vi "Joystick Outputs w Rumble.vi"(3 "Right Rumble":sgl, 4 "Left Rumble":sgl, 5 "JoystickDevRef":T1) -> (0 "POV":cluster{"POV":i16}, 1 "Axis":T3, 2 "Buttons":T4)   [LabVIEW 2020]
uses:
  <vilib>/Rock Robotics/WPI/Joystick/WPI_JoystickDevRef.ctl
  <vilib>/Rock Robotics/WPI/Joystick/WPI_JoystickDeviceEnum.ctl
panel:
  out "POV BL":bool
  out "POV BR":bool
  out "POV TR":bool
  out "POV TR":bool
  out "POV B":bool
  out "POV T":bool
  out "POV L":bool
  out "POV R":bool
  out "POV C":bool
  out "\"x' 13":bool
  out "\"x' 12":bool
  out "\"x' 11":bool
  out "\"x' 10":bool
  out "\"x' 9":bool
  out "\"x' 8":bool
  out "\"x' 7":bool
  out "\"x' 2":bool
  out "\"x' 6":bool
  out "\"x' 4":bool
  out "\"x' 3":bool
  out "\"x' 2":bool
  out "\"x'":bool
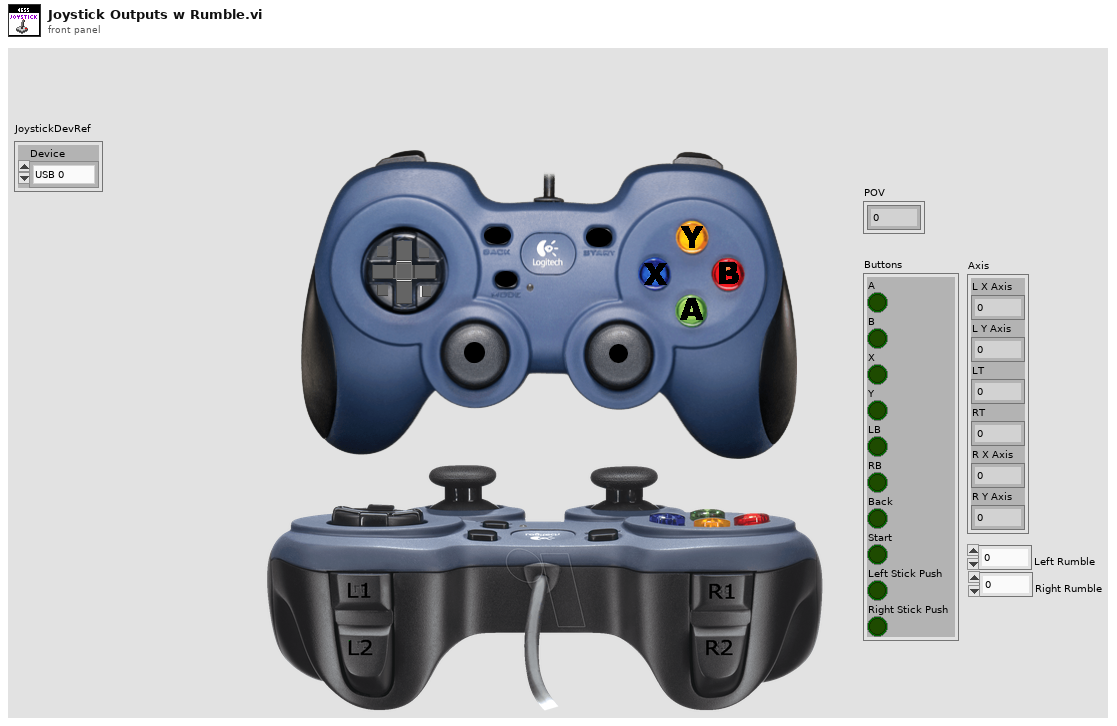
[diagram p1: front panel]
types:
  T1 = typedef "WPI_JoystickDevRef.ctl" = cluster{"Device":T2}
  T2 = typedef "WPI_JoystickDeviceEnum.ctl" = enum16{"USB 0", "USB 1", "USB 2", "USB 3", "USB 4", "USB 5"}
  T3 = cluster{"L X Axis":dbl, "L Y Axis":dbl, "LT":dbl, "RT":dbl, "R X Axis":dbl, "R Y Axis":dbl}
  T4 = cluster{"A":bool, "B":bool, "X":bool, "Y":bool, "LB":bool, "RB":bool, "Back":bool, "Start":bool, "Left Stick Push":bool, "Right Stick Push":bool}
  T5 = cluster{"Buttons[0]":bool, "Buttons[1]":bool, "Buttons[2]":bool, "Buttons[3]":bool, "Buttons[4]":bool, "Buttons[5]":bool, "Buttons[6]":bool, "Buttons[7]":bool, "Buttons[8]":bool, "Buttons[9]":bool}
  T6 = cluster{"Axes[0]":dbl, "Axes[1]":dbl, "Axes[2]":dbl, "Axes[3]":dbl, "Axes[4]":dbl, "Axes[5]":dbl}
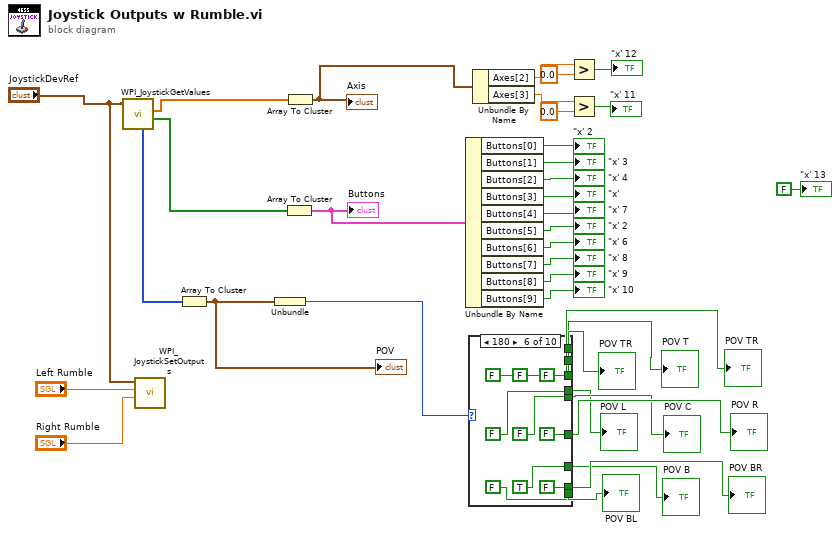
[diagram p0: block diagram]
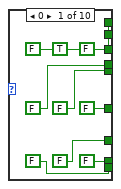
[diagram p2: hidden frame]
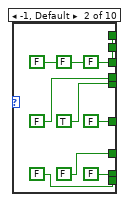
[diagram p3: hidden frame]
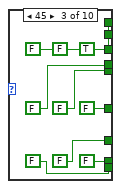
[diagram p4: hidden frame]
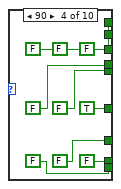
[diagram p5: hidden frame]
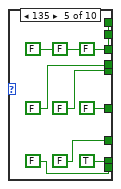
[diagram p6: hidden frame]
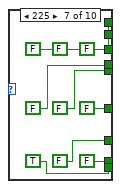
[diagram p7: hidden frame]
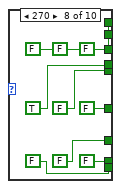
[diagram p8: hidden frame]
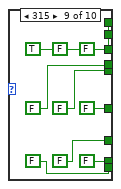
[diagram p9: hidden frame]
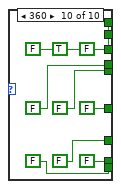
[diagram p10: hidden frame]
diagram:
  n1 = call <vilib>:"WPI_JoystickGetValues.vi"("JoystickDevRef"="JoystickDevRef") -> ("Buttons"=w36:bool[], "Axes"=w35:dbl[], "POVs"=w34:i16[])  [unwired: 6 in, 2 out]
  n2 = call <vilib>:"WPI_JoystickSetOutputs.vi"("Right Rumble"="Right Rumble", "Left Rumble"="Left Rumble", "JoystickDevRef"="JoystickDevRef") -> ()  [unwired: 7 in, 2 out]
  n3 = Array To Cluster(array=w34) -> (cluster=w16:cluster{"POVs[0]":i16})
  "POV" <- w16
  n4 = Unbundle(w16) -> ("POVs[0]"=w5:i16)
  n5 = Array To Cluster(array=w36) -> (cluster=w33:T5)
  "Buttons" <- w33
  n6 = Array To Cluster(array=w35) -> (cluster=w22:T6)
  "Axis" <- w22
  n7 = Unbundle By Name(w33) -> ("Buttons[0]"=→"\"x' 2":bool, "Buttons[1]"=→"\"x' 3":bool, "Buttons[2]"=→"\"x' 4":bool, "Buttons[3]"=→"\"x'":bool, "Buttons[4]"=→"\"x' 7":bool, "Buttons[5]"=→"\"x' 2":bool, "Buttons[6]"=→"\"x' 6":bool, "Buttons[7]"=→"\"x' 8":bool, "Buttons[8]"=→"\"x' 9":bool, "Buttons[9]"=→"\"x' 10":bool)
  n8 = case shown="180" w5 {
    tunnel: [FALSE ("POV TR") FALSE ("POV TR") FALSE ("POV TR") FALSE ("POV TR") FALSE ("POV TR") FALSE ("POV TR") FALSE ("POV TR") FALSE ("POV TR") TRUE ("POV TR") FALSE ("POV TR")] -> w14
    tunnel: [TRUE ("POV T") FALSE ("POV T") FALSE ("POV T") FALSE ("POV T") FALSE ("POV T") FALSE ("POV T") FALSE ("POV T") FALSE ("POV T") FALSE ("POV T") TRUE ("POV T")] -> w13
    tunnel: [FALSE ("POV TR") FALSE ("POV TR") TRUE ("POV TR") FALSE ("POV TR") FALSE ("POV TR") FALSE ("POV TR") FALSE ("POV TR") FALSE ("POV TR") FALSE ("POV TR") FALSE ("POV TR")] -> w12
    tunnel: [FALSE ("POV TR") FALSE ("POV TR") FALSE ("POV TR") TRUE ("POV TR") FALSE ("POV TR") FALSE ("POV TR") FALSE ("POV TR") FALSE ("POV TR") FALSE ("POV TR") FALSE ("POV TR")] -> w11
    tunnel: [FALSE ("POV T") TRUE ("POV T") FALSE ("POV T") FALSE ("POV T") FALSE ("POV T") FALSE ("POV T") FALSE ("POV T") FALSE ("POV T") FALSE ("POV T") FALSE ("POV T")] -> w10
    tunnel: [FALSE ("POV TR") FALSE ("POV TR") FALSE ("POV TR") FALSE ("POV TR") FALSE ("POV TR") FALSE ("POV TR") FALSE ("POV TR") TRUE ("POV TR") FALSE ("POV TR") FALSE ("POV TR")] -> w9
    tunnel: [FALSE ("POV TR") FALSE ("POV TR") FALSE ("POV TR") FALSE ("POV TR") TRUE ("POV TR") FALSE ("POV TR") FALSE ("POV TR") FALSE ("POV TR") FALSE ("POV TR") FALSE ("POV TR")] -> w8
    tunnel: [FALSE ("POV T") FALSE ("POV T") FALSE ("POV T") FALSE ("POV T") FALSE ("POV T") TRUE ("POV T") FALSE ("POV T") FALSE ("POV T") FALSE ("POV T") FALSE ("POV T")] -> w7
    tunnel: [FALSE ("POV TR") FALSE ("POV TR") FALSE ("POV TR") FALSE ("POV TR") FALSE ("POV TR") FALSE ("POV TR") TRUE ("POV TR") FALSE ("POV TR") FALSE ("POV TR") FALSE ("POV TR")] -> w6
    frame 0 {
    }
    frame -1, Default {
    }
    frame 45 {
    }
    frame 90 {
    }
    frame 135 {
    }
    frame 180 {
    }
    frame 225 {
    }
    frame 270 {
    }
    frame 315 {
    }
    frame 360 {
    }
  }
  "POV C" <- w10
  "POV R" <- w11
  "POV L" <- w9
  "POV T" <- w13
  "POV B" <- w7
  "POV TR" <- w12
  "POV TR" <- w14
  "POV BR" <- w8
  "POV BL" <- w6
  n9 = Unbundle By Name(w22) -> ("Axes[2]"=w21:dbl, "Axes[3]"=w20:dbl)
  n10 = Greater?(x=w21, y=0.0) -> (0:→"\"x' 12":bool)
  n11 = Greater?(x=w20, y=0.0) -> (0:→"\"x' 11":bool)
  "\"x' 13" <- FALSE ("\"x' 13")
